vi "READ ALL PYR ORNL Ver1.vi"() -> ()   [LabVIEW 2016]
uses:
  <vilib>/Platform/TimedLoop/XDataNode/timing_clust.ctl
  <vilib>/Platform/TimedLoop/XDataNode/nitl_modes.ctl
  <vilib>/Platform/TimedLoop/XDataNode/wakeup.ctl
  <vilib>/DAQmx/read.llb/DAQmx Read (Analog 1D DBL NChan 1Samp).vi
  <vilib>/DAQmx/miscellaneous.llb/DAQmx Fill In Error Info.vi
  <vilib>/platform/TimedLoop/XDataNode/XDataNode.xnode
  <vilib>/Platform/TimedLoop/XDataNode/XDNodeRunTimeDep.lvlib
panel:
  out "Pyrometers":dbl[](array[numeric])
  out "Working?":bool[](array[boolean])
  in  "stop":bool
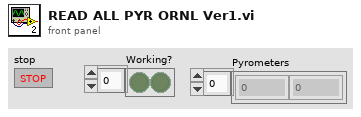
[diagram p1: front panel]
types:
  T1 = typedef "XDNodeRunTimeDep.lvlib/timing_clust.ctl" = cluster{"Expected End [f-1]":u64, "Actual End [f-1]":u64, "Finished Late? [f-1]":bool, "Expected End [i-1]":u64, "Actual End [i-1]":u64, "Finished Late? [i-1]":bool, "Expected Start [i]":u64, "Actual Start [i]":u64, "Expected Start [f]":u64, "Actual Start [f]":u64, "Source Name":string, "Structure Name":string, "Period":i64, "Deadline":i64, "Offset":i64, "Start":i64, "Priority":i32, "Timeout":i32, "Mode":T2, "Wakeup Reason":T3, "Error":errorcluster, "Source Type":string, "Secondary Source Type":string, "Global End Time":u64, "Global Start Time":u64, "Frame Duration":u64, "Iteration Duration":u64, "Assigned CPU":i32, "I/O Scan Engine Mode":u32}
  T2 = typedef "XDNodeRunTimeDep.lvlib/nitl_modes.ctl" = enum32{"No Change", "Process missed periods, maintain original phase", "Discard missed periods, maintain original phase", "Process missed periods, ignore original phase", "Discard missed periods, ignore original phase"}
  T3 = typedef "XDNodeRunTimeDep.lvlib/wakeup.ctl" = enum32{"Normal", "Aborted", "Asynchronous wakeup", "Timing source error", "Timed loop error", "Timeout"}
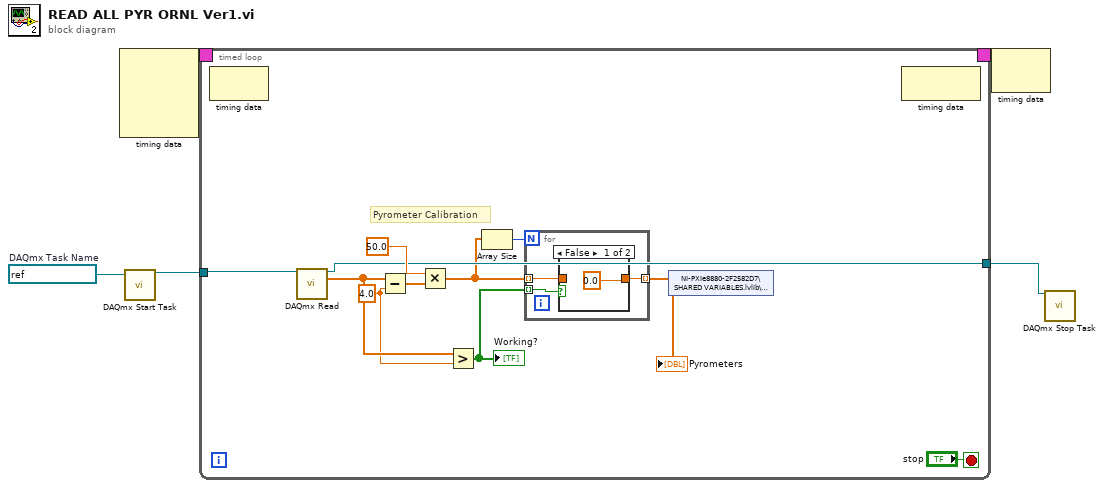
[diagram p0: block diagram]
diagram:
  w3 = refnum<k21> "Pyrometers"  # DAQmx Task Name
  n1 = node-c288() -> (w5:T1)  [unwired: 4 in]
  n2 = call <vilib>:"DAQmx Start Task.vi"("task/channels in"=w3) -> ("task out"=w2:refnum<k21>)  [unwired: 13 in, 1 out]
  n3 = timed-loop {
    timing: w5 -> [_]
    timing-out: [_] -> w4
    tunnel: w2 -> [w16]
    tunnel: [w12] -> w1
    stop <- "stop" stop-if-true
    w10 = 4.0 ("y")
    # "Pyrometer Calibration"
    n4 = node-c288() -> ()  [unwired: 1 in, 1 out]
    n5 = call-poly <vilib>:"DAQmx Read.vi"("task/channels in"=w16) -> ("task out"=w12:refnum<k21>, "data"=w11:dbl[])  [unwired: 12 in, 1 out]
    n6 = Subtract(x=w11, y=w10) -> (x-y=w15:dbl[])
    n7 = Multiply(x=50.0, y=w15) -> (x*y=w8:dbl[])
    n8 = Greater?(x=w11, y=w10) -> (0:w7:bool[])
    "Working?" <- w7
    n9 = Array Size(array=w8) -> (size(s)=w9:i32)
    n10 = for {
      N: w9 -> [_]
      tunnel: w8 -> [w18] mode=indexing
      tunnel: w7 -> [w19] mode=indexing
      tunnel: [w17] -> w6 mode=indexing
      n11 = case shown="False" w19 {
        tunnel: w18 -> [_ w21]
        tunnel: [0.0 w21] -> w17
        frame False {
        }
        frame True {
        }
      }
    }
    "Pyrometers" <- w6
    n12 = shared-variable "NI-PXIe8880-2F2582D7\\SHARED VARIABLES.lvlib\\Pyrometers"(w6) -> ()  [unwired: 1 in, 1 out]
    n13 = node-c288() -> ()  [unwired: 1 in, 1 out]
  }
  n14 = node-c288(w4) -> ()  [unwired: 1 out]
  n15 = call <vilib>:"DAQmx Stop Task.vi"("task/channels in"=w1) -> ()  [unwired: 13 in, 2 out]
